vi "Event Structure Loop with PanelClose Event.vi"   [LabVIEW 2017]
doc: "Use this VI as a template. This VI is a default template that handles user events when a VI needs to be shutdown."
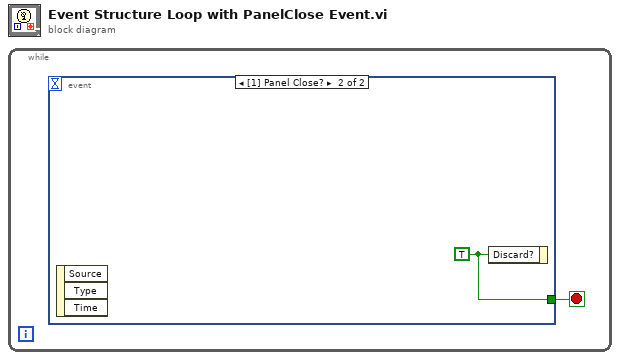
[diagram p0: block diagram]
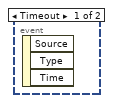
[diagram p2: hidden frame]
diagram:
  n1 = while {
    stop <- w1 stop-if-true
    n2 = event shown="[1] Panel Close?" {
      selector: _ -> [_ _]
      dyn-events: _ -> [_ _]
      timeout: _ -> [_ _]
      tunnel: [_ w2] -> w1
      event Timeout {
        n3 = event-data() -> ()  [unwired: 1 in, 3 out]
      }
      event Panel Close? {
        w2 = TRUE ("Discard?")
        n4 = event-data() -> ()  [unwired: 1 in, 3 out]
        n5 = event-data("Discard?"=w2) -> ()  [unwired: 1 in, 1 out]
      }
    }
  }
